vi "Append Call Chain.vi"(6 "Include Call Chain?":bool, 11 "Input String":string) -> (3 "Output String":string)   [LabVIEW 2021]
doc: "Appends a string containing call chain of the VI with two levels removed."
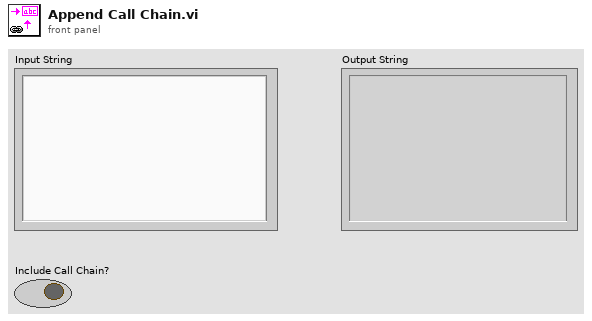
[diagram p1: front panel]
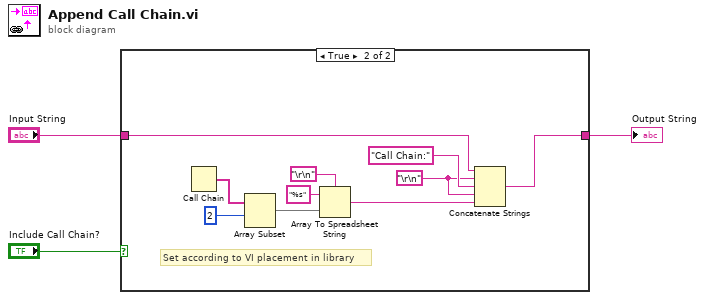
[diagram p0: block diagram]
diagram:
  n1 = case shown="True" "Include Call Chain?" {
    tunnel: "Input String" -> [w4 w6]
    tunnel: [w4 w5] -> w2
    frame False {
    }
    frame True {
      w7 = "\r\n"
      # "Set according to VI placement in library"
      n2 = Call Chain() -> (call chain=w14:string[])
      n3 = Array Subset(array=w14, index=2) -> (w12:string[])  [unwired: 1 in]
      n4 = Array To Spreadsheet String(delimiter (Tab)="\r\n", array=w12, 3:"%s" ("format string")) -> (spreadsheet string=w10:string)
      n5 = Concatenate Strings(w6, w7, "Call Chain:", w7, w10) -> (w5:string)
    }
  }
  "Output String" <- w2
